vi "PathPlanner_PathSegment_Resolution.vi"() -> (3 "Resolution":dbl=0.05)   [LabVIEW 2019, in "PathPlanner24.lvlib"]
doc: "The resolution used during path generation\n\nOutputs:\n - Resolution - double"
uses:
  PathPlanner24.lvlib
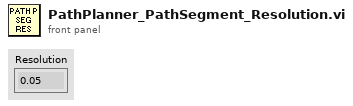
[diagram p1: front panel]
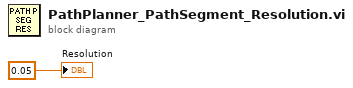
[diagram p0: block diagram]
diagram:
  "Resolution" <- 0.05
